vi "写入参数.vi"(7 "写入参数":T1(ring), 8 "error in (no error)":errorcluster, 11 "写入值":sgl) -> (0 "error out":errorcluster)   [LabVIEW 2016, in "一代CodMn.lvlib"]
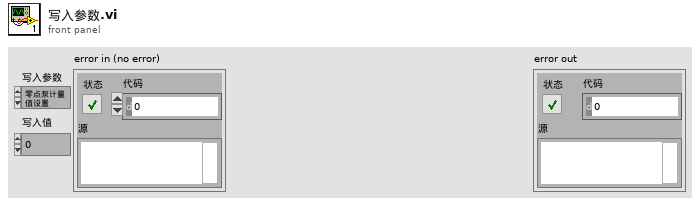
[diagram p1: front panel]
types:
  T1 = enum16{"零点泵计量值设置", "零点滴定值设置", "标度泵计量值设置", "标度滴定值设定", "标液浓度设置"}
  T2 = enum16{"open", "close", "readHR", "writeHR", "readCoil", "writeCoil"}
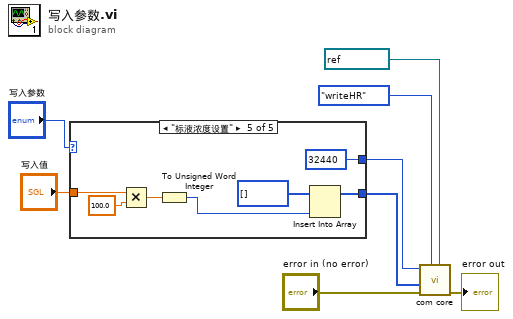
[diagram p0: block diagram]
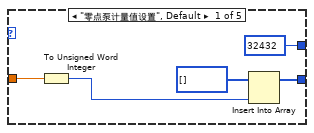
[diagram p2: hidden frame]
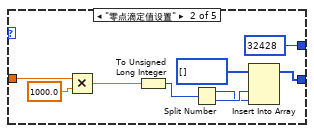
[diagram p3: hidden frame]
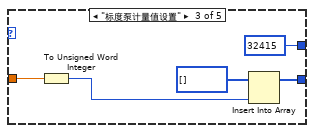
[diagram p4: hidden frame]
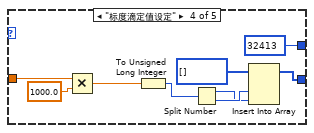
[diagram p5: hidden frame]
diagram:
  n1 = case shown="\"标液浓度设置\"" "写入参数" {
    tunnel: [u16 32432 ("starting address") u16 32428 ("starting address") u16 32415 ("starting address") u16 32413 ("starting address") u16 32440 ("starting address")] -> w6
    tunnel: "写入值" -> [w12 w21 w25 w29 w39]
    tunnel: [w9 w16 w24 w28 w40] -> w4
    frame "零点泵计量值设置", Default {
      n2 = To Unsigned Word Integer(number=w12) -> (unsigned 16bit integer=w10:u16)
      n3 = Insert Into Array(array=u16[] [] ("HR values"), new element=w10) -> (w9:u16[])  [unwired: 1 in]
    }
    frame "零点滴定值设置" {
      n4 = Multiply(x=w21, y=sgl 1000.0) -> (x*y=w19:sgl)
      n5 = To Unsigned Long Integer(number=w19) -> (unsigned 32bit integer=w18:u32)
      n6 = Split Number(x=w18) -> (hi(x)=w14:u16, lo(x)=w15:u16)
      n7 = Insert Into Array(array=u16[] [] ("HR values"), new element #1=w15, new element #2=w14) -> (w16:u16[])  [unwired: 1 in]
    }
    frame "标度泵计量值设置" {
      n8 = To Unsigned Word Integer(number=w25) -> (unsigned 16bit integer=w26:u16)
      n9 = Insert Into Array(array=u16[] [] ("HR values"), new element=w26) -> (w24:u16[])  [unwired: 1 in]
    }
    frame "标度滴定值设定" {
      n10 = Multiply(x=w29, y=sgl 1000.0) -> (x*y=w34:sgl)
      n11 = To Unsigned Long Integer(number=w34) -> (unsigned 32bit integer=w33:u32)
      n12 = Split Number(x=w33) -> (hi(x)=w30:u16, lo(x)=w31:u16)
      n13 = Insert Into Array(array=u16[] [] ("HR values"), new element #1=w31, new element #2=w30) -> (w28:u16[])  [unwired: 1 in]
    }
    frame "标液浓度设置" {
      n14 = Multiply(x=w39, y=sgl 100.0) -> (x*y=w38:sgl)
      n15 = To Unsigned Word Integer(number=w38) -> (unsigned 16bit integer=w37:u16)
      n16 = Insert Into Array(array=u16[] [] ("HR values"), new element=w37) -> (w40:u16[])  [unwired: 1 in]
    }
  }
  n17 = call "com core.vi"("VISA Resource"=refnum<visa-resource-name> "COM3", "功能"=T2."writeHR", "error in (no error)"="error in (no error)", "HR values"=w4, "starting address"=w6) -> ("error out"=→"error out":errorcluster)  [unwired: 4 in, 2 out]
